vi "Read Step Config Class.vi"(8 "error in (no error)":errorcluster, 11 "StepNode in":refnum<class "StepNode.lvclass">) -> (0 "error out":errorcluster, 2 "Step Config.lvclass":refnum<class "Step Config.lvclass">, 3 "StepNode out":refnum<class "StepNode.lvclass">)   [LabVIEW 2015, in "StepNode.lvclass"]
uses:
  StepNode.lvclass
  Prototype/classes/Step/Config/Step Config.lvclass
  StepNode.lvclass/StepNode.ctl
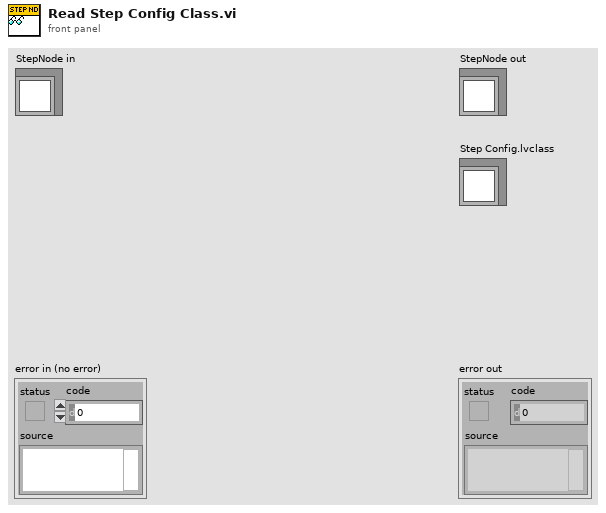
[diagram p1: front panel]
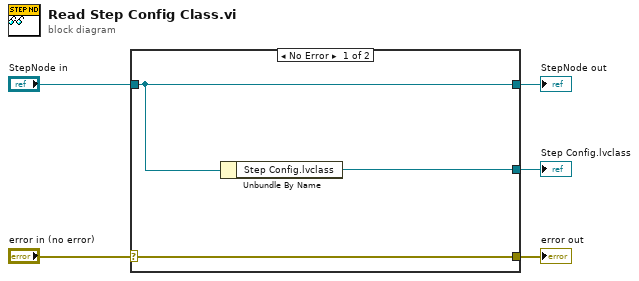
[diagram p0: block diagram]
diagram:
  n1 = case shown="No Error" "error in (no error)" {
    selector: "error in (no error)" -> [w8 w9]
    tunnel: [w8 w9] -> w4
    tunnel: [w7 w10] -> w2
    tunnel: "StepNode in" -> [w7 w10]
    tunnel: [w6 _] -> w1
    frame No Error {
      n2 = Unbundle By Name(w7) -> ("Step Config.lvclass"=w6:refnum<class "Step Config.lvclass">)
    }
    frame Error {
    }
  }
  "error out" <- w4
  "StepNode out" <- w2
  "Step Config.lvclass" <- w1
